vi "Configure FFT Average.vi"(8 "error in (no error)":errorcluster, 10 "FFT Waveform Count (8: 8)":i32=8, 11 "VISA resource name":refnum<visa-resource-name>) -> (0 "error out":errorcluster, 3 "VISA resource name out":refnum<visa-resource-name>)   [LabVIEW 2015, in "Agilent 2000 3000 X-Series.lvlib"]
doc: "Sets the number of waveforms to be averaged together.\n\nNotes:\nOnly applicable for 3000 T, 3000G Series. \nThe FFT subsystem controls the FFT function in the oscilloscope."
uses:
  Agilent 2000 3000 X-Series.lvlib
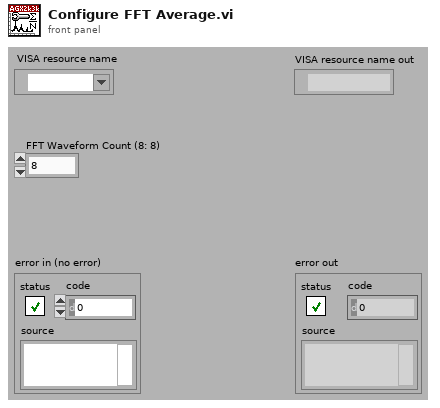
[diagram p1: front panel]
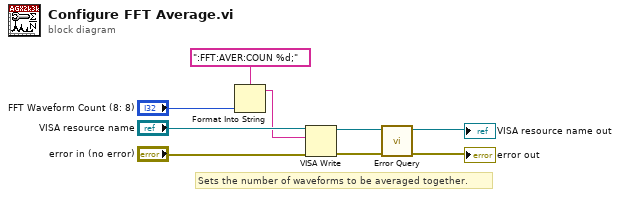
[diagram p0: block diagram]
diagram:
  # "Sets the number of waveforms to be averaged together."
  n1 = Format Into String(format string=":FFT:AVER:COUN %d;", "FFT Waveform Count (8: 8)") -> (resulting string=w4:string)  [unwired: 2 in, 1 out]
  n2 = VISA Write(VISA resource name="VISA resource name", write buffer=w4, error in (no error)="error in (no error)") -> (VISA resource name out=w8:refnum<visa-resource-name>, error out=w7:errorcluster)  [unwired: 1 out]
  n3 = call "Error Query.vi"("error in (no error)"=w7, "VISA resource name"=w8) -> ("error out"=→"error out":errorcluster, "VISA resource name out"=→"VISA resource name out":refnum<visa-resource-name>)  [unwired: 8 out]
